vi "UHR-Fleezers Control (host) - 11.9c.vi"() -> ()   [LabVIEW 2014] (continued)
                  n307 = local read "Y RF Frequency Limits (MHz)"() -> (w501:T17)
                  n308 = local read "X RF Frequency Limits (MHz)"() -> (w502:T17)
                  n309 = local read "BD 2 Frequency 2 (MHz)"() -> (w508:dbl)
                  n310 = local read "BD 2 Frequency 3 (MHz)"() -> (w507:dbl)
                  n311 = local read "BD 1 Frequency 3 (MHz)"() -> (w509:dbl)
                  n312 = call "set RF board frequency - interlace.vi"("Board 2 Frequency Limits"=w501, "Board 1 Frequency Limits"=w502, "FPGA VI Reference In"=w494, "Board 2 Frequency 3 (MHz)"=w507, "Board 1 Frequency 3 (MHz)"=w509, "Board 2 Frequency 2 (MHz)"=w508, "Board 2 Frequency 1 (MHz)"=w505, "Board 1 Frequency 2 (MHz)"=w495, "Board 1 Frequency 1  (MHz)"=w506) -> ()  [unwired: 1 in, 2 out]
                }
                frame #1 {
                  n313 = And(x=w559, y=w556) -> (x .and. y?=w558:bool)
                  n314 = case "Only if were fishing and now formed tether" shown="True" w558 {
                    tunnel: w557 -> [w561 w576]
                    tunnel: [w560 w575] -> w555
                    tunnel: w554 -> [_ w571]
                    frame False {
                      n315 = local read "Fish"() -> (w560:bool)
                      n316 = case shown="False" w560 {
                        tunnel: w561 -> [w562 _]
                        frame False {
                          n317 = property on="BD 1 Frequency 1 (MHz)" class="DigNum (strict)"("Val(Sgnl)"=w562) -> ()  [unwired: 2 in, 2 out]
                        }
                        frame True {
                        }
                      }
                    }
                    frame True {
                      w575 = FALSE ("Fish for Tether")
                      n318 = call <vilib>:"Beep.vi"() -> ()  [unwired: 3 in, 9 out]
                      n319 = Number To Decimal String(number=w571, width (-)=i16 1) -> (decimal integer string=w569:string)
                      n320 = Concatenate Strings("Formed tether in ", w569, " attempt(s)." ("string")) -> (w566:string)
                      n321 = local read "Messages"() -> (w573:string)
                      n322 = local write "Fish"(w575) -> ()
                      n323 = call "Update messages.vi"("Message to add"=w566, "Old message string"=w573) -> ("New message string"=w572:string)
                      n324 = local write "Messages"(w572) -> ()
                      n325 = Get Date/Time In Seconds() -> (seconds since 1Jan1904=→"Time tether formed":timestamp)
                      n326 = local read "Flow ON\nduring cal?"() -> (w563:bool)
                      n327 = property on="Sample Channel\nFlow" class="Bool (strict)"("Val(Sgnl)"=w563) -> (error out=w564:errorcluster)  [unwired: 2 in, 1 out]
                      n328 = case shown="\"2\", \"3\", \"4\", \"5\", \"6\"" "Then..." {
                        selector: "Then..." -> [_ w579 _ _]
                        tunnel: w576 -> [w578 _ _ _]
                        tunnel: w564 -> [_ _ _ _]
                        frame "1", Default {
                          n329 = property on="BD 1 Frequency 1 (MHz)" class="DigNum (strict)"("Val(Sgnl)"=w578) -> ()  [unwired: 2 in, 2 out]
                        }
                        frame "2", "3", "4", "5", "6" {
                          n330 = flat-sequence {
                            tunnel: w579 -> [w585]
                            frame #0 {
                              n331 = local read "Flow ON\nduring cal?"() -> (w580:bool)
                              n332 = property on="Sample Channel\nFlow" class="Bool (strict)"("Val(Sgnl)"=w580) -> ()  [unwired: 2 in, 2 out]
                              n333 = property on="Trap D (MHz)" class="DigNum (strict)"("Val(Sgnl)"="Move to D 1 (MHz)") -> ()  [unwired: 2 in, 2 out]
                            }
                            frame #1 {
                              n334 = local read "Wait Before Save (s)"() -> (w582:u32)
                              n335 = Multiply(x=u32 1000 ("milliseconds to wait"), y=w582) -> (x*y=w584:u32)
                              n336 = Wait (ms)(milliseconds to wait=w584) -> ()  [unwired: 1 out]
                            }
                            frame #2 {
                              n337 = case shown="\"5\", \"6\"" w585 {
                                selector: w585 -> [w588 w598 _]
                                frame "3", "4" {
                                n338 = flat-sequence {
                                tunnel: w588 -> [w589]
                                tunnel: [w589] -> w586
                                tunnel: [w591] -> w587
                                tunnel: w586 -> [w591]
                                tunnel: w587 -> [w595]
                                frame #0 {
                                n339 = property on="Green ON/Interlacing" class="Bool (strict)"("Val(Sgnl)"=TRUE ("Value (Signaling)")) -> ()  [unwired: 2 in, 2 out]
                                }
                                frame #1 {
                                n340 = Multiply(x="Wait Before Save (s)", y=u32 1000 ("x")) -> (x*y=w593:u32)
                                n341 = Wait (ms)(milliseconds to wait=w593) -> ()  [unwired: 1 out]
                                }
                                frame #2 {
                                n342 = property on="Start Saving" class="Bool (strict)"("Value"=TRUE ("Start Saving")) -> ()  [unwired: 2 in, 2 out]
                                n343 = case shown="\"4\"" w595 {
                                frame Default {
                                }
                                frame "4" {
                                n344 = property on="Fl. Triggered..." class="Bool (strict)"("Val(Sgnl)"=TRUE ("Value (Signaling)")) -> ()  [unwired: 2 in, 2 out]
                                }
                                }
                                }
                                }
                                }
                                frame "5", "6" {
                                n345 = stacked-sequence {
                                tunnel: w598 -> [_ _ _ _ _ _ w610]
                                frame #0 {
                                n346 = Replace Array Subset(array=u32[] [0] ("Index Values"), new element="Raster Set\nUpon Tether", index=0) -> (w599:u32[])
                                n347 = property on="Saved AOD Raster Scan Parameter Sets" class="Arr (strict)"("Index Values"=w599) -> ()  [unwired: 2 in, 2 out]
                                }
                                frame #1 {
                                n348 = Wait (ms)(milliseconds to wait=u32 500) -> ()  [unwired: 1 out]
                                }
                                frame #2 {
                                n349 = property on="Load parameters" class="Bool (strict)"("Val(Sgnl)"=TRUE ("Value (Signaling)")) -> ()  [unwired: 2 in, 2 out]
                                n350 = case shown="True" "Green ON during\nraster?" {
                                frame False {
                                }
                                frame True {
                                n351 = property on="Green ON/Interlacing" class="Bool (strict)"("Val(Sgnl)"=TRUE ("Value (Signaling)")) -> ()  [unwired: 2 in, 2 out]
                                }
                                }
                                }
                                frame #3 {
                                n352 = Wait (ms)(milliseconds to wait=u32 500) -> ()  [unwired: 1 out]
                                }
                                frame #4 {
                                n353 = property on="Trap Raster Scan" class="Bool (strict)"("Val(Sgnl)"=TRUE ("Value (Signaling)")) -> ()  [unwired: 2 in, 2 out]
                                }
                                frame #5 {
                                n354 = Wait (ms)(milliseconds to wait=u32 2000) -> ()  [unwired: 1 out]
                                }
                                frame #6 {
                                n355 = flat-sequence {
                                tunnel: w610 -> [w617]
                                frame #0 {
                                n356 = while {
                                stop <- w613 stop-if-true
                                n357 = local read "Raster Scanning..."() -> (w612:bool)
                                n358 = local read "Saving..."() -> (w615:bool)
                                n359 = Wait (ms)(milliseconds to wait=u32 100) -> ()  [unwired: 1 out]
                                n360 = Not(x=w615) -> (.not. x?=w614:bool)
                                n361 = Not(x=w612) -> (.not. x?=w611:bool)
                                n362 = And(x=w614, y=w611) -> (x .and. y?=w613:bool)
                                }
                                }
                                frame #1 {
                                n363 = local read "Tether"() -> (w618:bool)
                                n364 = case shown="True" w618 {
                                tunnel: w617 -> [_ w620]
                                frame False {
                                n365 = property on="Fish" class="Bool (strict)"("Val(Sgnl)"="Fish again after \nraster break?") -> ()  [unwired: 2 in, 2 out]
                                }
                                frame True {
                                n366 = stacked-sequence {
                                tunnel: w620 -> [_ w624 _ _ _ _ _ _]
                                frame #0 {
                                n367 = property on="Trap D (MHz)" class="DigNum (strict)"("Val(Sgnl)"="Move to D 2 (MHz)") -> ()  [unwired: 2 in, 2 out]
                                n368 = case shown="True" "Flow ON after\ntether testing?" {
                                frame False {
                                }
                                frame True {
                                n369 = property on="Sample Channel\nFlow" class="Bool (strict)"("Val(Sgnl)"=TRUE ("Value (Signaling)")) -> ()  [unwired: 2 in, 2 out]
                                }
                                }
                                }
                                frame #1 {
                                n370 = flat-sequence {
                                tunnel: w624 -> [w625]
                                frame #0 {
                                n371 = case shown="\"6\"" w625 {
                                frame Default {
                                }
                                frame "6" {
                                n372 = flat-sequence {
                                frame #0 {
                                n373 = Wait (ms)(milliseconds to wait=u32 500) -> ()  [unwired: 1 out]
                                }
                                frame #1 {
                                n374 = property on="Green ON/Interlacing" class="Bool (strict)"("Val(Sgnl)"=TRUE ("Green Laser ON/Interlacing")) -> ()  [unwired: 2 in, 2 out]
                                }
                                }
                                }
                                }
                                }
                                frame #1 {
                                n375 = case shown="True" "Save at end (5, 6)" {
                                selector: "Save at end (5, 6)" -> [_ w629]
                                frame False {
                                }
                                frame True {
                                n376 = flat-sequence {
                                tunnel: w629 -> [w631]
                                frame #0 {
                                n377 = Wait (ms)(milliseconds to wait=u32 500) -> ()  [unwired: 1 out]
                                }
                                frame #1 {
                                n378 = local write "Start Saving"(w631) -> ()
                                }
                                }
                                }
                                }
                                }
                                }
                                }
                                frame #2 {
                                n379 = local read "Bead Sep. Int. Time (s)"() -> (w634:dbl)
                                n380 = Multiply(x=w634, y=1000.0) -> (x*y=w633:dbl)
                                n381 = Wait (ms)(milliseconds to wait=w633) -> ()  [unwired: 1 out]
                                }
                                frame #3 {
                                n382 = property on="Remove Offset" class="Bool (strict)"("Val(Sgnl)"=TRUE ("Value (Signaling)")) -> ()  [unwired: 2 in, 2 out]
                                }
                                frame #4 {
                                n383 = property on="Read FX file" class="Bool (strict)"("Val(Sgnl)"=TRUE ("Value (Signaling)")) -> ()  [unwired: 2 in, 2 out]
                                }
                                frame #5 {
                                n384 = Wait (ms)(milliseconds to wait=u32 300) -> ()  [unwired: 1 out]
                                }
                                frame #6 {
                                n385 = local read "Bad fit error"() -> (w643:dbl)
                                n386 = local read "Fit offset"() -> (w646:dbl)
                                n387 = Greater Or Equal?(x=w643, y="Bad fit thresh") -> (x >= y?=→"Bad fit":bool)
                                n388 = Greater Or Equal?(x=w646, y="Fit offset thresh") -> (x >= y?=→"Multiple tether":bool)
                                n389 = local read "Hyst. error"() -> (w640:dbl)
                                n390 = Greater Or Equal?(x=w640, y="Hysteresis thresh") -> (x >= y?=→"Hysteresis":bool)
                                }
                                frame #7 {
                                w651 = 0
                                n391 = local read "Bad fit error"() -> (w653:dbl)
                                n392 = local read "Hyst. error"() -> (w652:dbl)
                                n393 = local read "Fit offset"() -> (w654:dbl)
                                n394 = local read "Multiple tether"() -> (w660:bool)
                                n395 = local read "Hysteresis"() -> (w658:bool)
                                n396 = local read "Bad fit"() -> (w659:bool)
                                n397 = Not(x=w658) -> (.not. x?=w650:bool)
                                n398 = Not(x=w659) -> (.not. x?=w656:bool)
                                n399 = Greater?(x=w654, y=w651) -> (0:w649:bool)
                                n400 = Greater?(x=w653, y=w651) -> (0:w648:bool)
                                n401 = Greater?(x=w652, y=w651) -> (0:w647:bool)
                                n402 = Not(x=w660) -> (.not. x?=w657:bool)
                                n403 = Compound Arithmetic op=AND(w657, w656, w650, w649, w648, w647) -> (w655:bool)
                                "Good tether" <- w655
                                n404 = case shown="True" w655 {
                                frame False {
                                }
                                frame True {
                                n405 = call <vilib>:"Beep.vi"("use system alert? (T)"=FALSE, "duration (msec)"=u32 200, "frequency (Hz)"=u32 2000) -> ()  [unwired: 9 in]
                                }
                                }
                                }
                                }
                                }
                                }
                                }
                                }
                                }
                                }
                                }
                                frame "2", Default {
                                }
                              }
                            }
                            frame #3 {
                              n406 = local read "Multiple tether"() -> (w666:bool)
                              n407 = And(x="Break multiple", y=w666) -> (x .and. y?=w664:bool)
                              n408 = case shown="True" w664 {
                                frame False {
                                }
                                frame True {
                                n409 = stacked-sequence {
                                frame #0 {
                                n410 = property on="Trap D (MHz)" class="DigNum (strict)"("Val(Sgnl)"="Trap D to \nbreak (MHz)") -> ()  [unwired: 2 in, 2 out]
                                }
                                frame #1 {
                                n411 = case shown="True" "Fish after\nmultiple break" {
                                frame False {
                                }
                                frame True {
                                n412 = while {
                                stop <- w671 stop-if-true
                                n413 = local read "Multiple tether"() -> (w673:bool)
                                n414 = local read "Fish"() -> (w670:bool)
                                n415 = local read "Stop All"() -> (w669:bool)
                                n416 = Wait (ms)(milliseconds to wait=u32 100) -> ()  [unwired: 1 out]
                                n417 = Not(x=w673) -> (.not. x?=w672:bool)
                                n418 = Compound Arithmetic op=OR(w669, w672, w670) -> (w671:bool)
                                }
                                }
                                }
                                }
                                frame #2 {
                                n419 = local read "Fish after\nmultiple break"() -> (w678:bool)
                                n420 = local read "Stage Moving"() -> (w677:bool)
                                n421 = Not(x=w677) -> (.not. x?=w675:bool)
                                n422 = And(x=w678, y=w675) -> (x .and. y?=w676:bool)
                                n423 = property on="Fish" class="Bool (strict)"("Val(Sgnl)"=w676) -> ()  [unwired: 2 in, 2 out]
                                }
                                }
                                }
                              }
                            }
                            frame #4 {
                              n424 = local read "Bad fit"() -> (w680:bool)
                              n425 = And(x="Break bad fit", y=w680) -> (x .and. y?=w679:bool)
                              n426 = case shown="True" w679 {
                                frame False {
                                }
                                frame True {
                                n427 = stacked-sequence {
                                frame #0 {
                                n428 = local read "Trap D to \nbreak (MHz)"() -> (w682:dbl)
                                n429 = property on="Trap D (MHz)" class="DigNum (strict)"("Val(Sgnl)"=w682) -> ()  [unwired: 2 in, 2 out]
                                }
                                frame #1 {
                                n430 = case shown="True" "Fish after\nbad fit break?" {
                                frame False {
                                }
                                frame True {
                                n431 = while {
                                stop <- w686 stop-if-true
                                n432 = local read "Stop All"() -> (w684:bool)
                                n433 = local read "Bad fit"() -> (w685:bool)
                                n434 = local read "Fish"() -> (w687:bool)
                                n435 = Not(x=w685) -> (.not. x?=w688:bool)
                                n436 = Wait (ms)(milliseconds to wait=u32 100) -> ()  [unwired: 1 out]
                                n437 = Compound Arithmetic op=OR(w684, w688, w687) -> (w686:bool)
                                }
                                }
                                }
                                }
                                frame #2 {
                                n438 = local read "Fish after\nbad fit break?"() -> (w690:bool)
                                n439 = local read "Stage Moving"() -> (w693:bool)
                                n440 = Not(x=w693) -> (.not. x?=w692:bool)
                                n441 = And(x=w690, y=w692) -> (x .and. y?=w691:bool)
                                n442 = property on="Fish" class="Bool (strict)"("Val(Sgnl)"=w691) -> ()  [unwired: 2 in, 2 out]
                                }
                                }
                                }
                              }
                            }
                            frame #5 {
                              n443 = local read "Hysteresis"() -> (w695:bool)
                              n444 = And(x="Break hyst", y=w695) -> (x .and. y?=w694:bool)
                              n445 = case shown="True" w694 {
                                frame False {
                                }
                                frame True {
                                n446 = stacked-sequence {
                                frame #0 {
                                n447 = local read "Trap D to \nbreak (MHz)"() -> (w697:dbl)
                                n448 = property on="Trap D (MHz)" class="DigNum (strict)"("Val(Sgnl)"=w697) -> ()  [unwired: 2 in, 2 out]
                                }
                                frame #1 {
                                n449 = case shown="True" "Fish ater hyst?" {
                                frame False {
                                }
                                frame True {
                                n450 = while {
                                stop <- w703 stop-if-true
                                n451 = local read "Hysteresis"() -> (w702:bool)
                                n452 = local read "Stop All"() -> (w699:bool)
                                n453 = local read "Fish"() -> (w700:bool)
                                n454 = Wait (ms)(milliseconds to wait=u32 100) -> ()  [unwired: 1 out]
                                n455 = Not(x=w702) -> (.not. x?=w701:bool)
                                n456 = Compound Arithmetic op=OR(w699, w701, w700) -> (w703:bool)
                                }
                                }
                                }
                                }
                                frame #2 {
                                n457 = local read "Fish ater hyst?"() -> (w708:bool)
                                n458 = local read "Stage Moving"() -> (w707:bool)
                                n459 = Not(x=w707) -> (.not. x?=w706:bool)
                                n460 = And(x=w708, y=w706) -> (x .and. y?=w705:bool)
                                n461 = property on="Fish" class="Bool (strict)"("Val(Sgnl)"=w705) -> ()  [unwired: 2 in, 2 out]
                                }
                                }
                                }
                              }
                            }
                            frame #6 {
                              n462 = local read "Good tether"() -> (w709:bool)
                              n463 = case shown="True" w709 {
                                frame False {
                                }
                                frame True {
                                n464 = case shown="\"1\"" "If good, then:" {
                                frame "0", Default {
                                }
                                frame "1" {
                                n465 = property on="Force FB Script" class="Bool (strict)"("Val(Sgnl)"=TRUE ("Value (Signaling)")) -> ()  [unwired: 2 in, 2 out]
                                }
                                }
                                }
                              }
                            }
                          }
                        }
                        frame "7" {
                          n466 = property on="Force FB Script" class="Bool (strict)"("Val(Sgnl)"=TRUE ("Value (Signaling)")) -> ()  [unwired: 2 in, 2 out]
                        }
                        frame "8" {
                          n467 = property on="Fixed Traps Script" class="Bool (strict)"("Val(Sgnl)"=TRUE ("Value (Signaling)")) -> ()  [unwired: 2 in, 2 out]
                        }
                      }
                      "Tether" <- "Tether Alarm?"
                    }
                  }
                }
                frame #2 {
                  n468 = local read "Oscillate Set 1"() -> (w719:bool)
                  n469 = local read "Stop All"() -> (w717:bool)
                  n470 = Or(x=w719, y=w714) -> (x .or. y?=w716:bool)
                  n471 = Not(x=w716) -> (.not. x?=w718:bool)
                  n472 = Compound Arithmetic op=OR(w717, w718) -> (w715:bool)
                }
              }
              n473 = node-c288() -> ()  [unwired: 2 out]
            }
            n474 = node-c288(w469) -> ()  [unwired: 1 out]
          }
        }
      }
      event "Fl. Triggered...": Value Change {
        n475 = event-data() -> ()  [unwired: 7 out]
        n476 = case shown="True" "Fl. Triggered..." {
          frame False {
          }
          frame True {
            n477 = node-c288() -> (w730:T22)  [unwired: 4 out]
            n478 = timed-loop {
              timing: w730 -> [_]
              timing-out: [_] -> w729
              tunnel: "Action" -> [w738]
              shift-right: [w735] -> _
              shift-left: u8 255 -> [w737]
              shift-right: [w732] -> _
              shift-left: 255 -> [w734]
              stop <- w731 stop-if-true
              # "Reset confocal spot"
              n479 = node-c288() -> ()  [unwired: 2 out]
              n480 = flat-sequence {
                tunnel: w738 -> [w758]
                tunnel: w737 -> [w757]
                tunnel: [w756] -> w736
                tunnel: w734 -> [w743]
                tunnel: [w742] -> w733
                tunnel: [w1142] -> w731
                tunnel: w736 -> [w1141]
                tunnel: [w1141] -> w735
                tunnel: [w1140] -> w732
                tunnel: w733 -> [w1140]
                frame #0 {
                  n481 = local read "Delta Fl. 2"() -> (w755:dbl)
                  n482 = local read "Delta Fl. 1"() -> (w750:dbl)
                  n483 = Multiply(x="Fl. D Thresh. (kHz)", y=1000.0) -> (x*y=w745:dbl)
                  n484 = Select(t=w750, s="APD to Watch", f=w755) -> (s? t:f=w746:dbl)
                  n485 = Greater?(x=w746, y=w745) -> (0:w751:bool)
                  n486 = Or(x="Force Yank", y=w751) -> (x .or. y?=w749:bool)
                  n487 = And(x=w749, y="Yank when?") -> (x .and. y?=w747:bool)
                  n488 = case shown="False" w747 {
                    tunnel: w758 -> [w761 w964]
                    tunnel: w757 -> [w763 w960]
                    tunnel: [w763 w958] -> w756
                    tunnel: w746 -> [w769 _]
                    tunnel: w745 -> [w768 _]
                    tunnel: "Force Yank" -> [w766 _]
                    tunnel: w743 -> [w765 w957]
                    tunnel: [w764 w957] -> w742
                    frame False {
                      n489 = Negate(x=w768) -> (-x=w760:dbl)
                      n490 = local write "Fl. High"(TRUE ("Fl. High")) -> ()
                      n491 = Less?(x=w769, y=w760) -> (x < y?=w767:bool)
                      n492 = Or(x=w766, y=w767) -> (x .or. y?=w762:bool)
                      n493 = case shown="True" w762 {
                        tunnel: w765 -> [w770 w780]
                        tunnel: [w770 w779] -> w764
                        tunnel: w761 -> [_ w778]
                        frame False {
                        }
                        frame True {
                          n494 = flat-sequence {
                            tunnel: w780 -> [w786]
                            tunnel: w778 -> [w783]
                            tunnel: [w785] -> w777
                            tunnel: [w784] -> w776
                            tunnel: [w783] -> w775
                            tunnel: w774 -> [w782]
                            tunnel: [w782] -> w773
                            tunnel: w772 -> [w781]
                            tunnel: [w781] -> w771
                            tunnel: [w858] -> w779
                            tunnel: w777 -> [w858]
                            tunnel: w776 -> [w857]
                            tunnel: w775 -> [w856]
                            tunnel: w773 -> [w855]
                            tunnel: w771 -> [w854]
                            frame #0 {
                              n495 = call <vilib>:"Beep.vi"() -> ()  [unwired: 12 in]
                              n496 = local write "Waiting"(FALSE ("Waiting")) -> ()
                              n497 = Increment(x=w786) -> (x+1=w785:i32)
                              n498 = case shown="\"Yank\"" w783 {
                                tunnel: w785 -> [_ w791 _]
                                frame "Alarm", Default {
                                }
                                frame "Yank" {
                                n499 = flat-sequence {
                                tunnel: w791 -> [w794]
                                tunnel: [w793] -> w790
                                tunnel: [w792] -> w789
                                tunnel: w790 -> [w804]
                                tunnel: w789 -> [w805]
                                frame #0 {
                                n500 = local read "Yank Delay (s)"() -> (w797:dbl)
                                n501 = local read "N Array El"() -> (w792:u8)
                                n502 = Quotient & Remainder(x=w794, y=w792) -> (x-y*floor(x/y)=w793:i32)  [unwired: 1 out]
                                n503 = Multiply(x=w797, y=1000.0) -> (x*y=w795:dbl)
                                n504 = Wait (ms)(milliseconds to wait=w795) -> ()  [unwired: 1 out]
                                }
                                frame #1 {
                                n505 = local read "Yank to which?"() -> (w799:bool)
                                n506 = local read "Random Choice"() -> (w809:bool)
                                n507 = local read "Yank to Trap D (MHz)"() -> (w802:dbl[])
                                n508 = local read "Yank to SP"() -> (w803:dbl[])
                                n509 = Random Number (0-1)() -> (number: 0 to 1=w808:dbl)
                                n510 = Multiply(x=w805, y=w808) -> (x*y=w807:dbl)
                                n511 = Round Toward -Infinity(1:w807) -> (0:w806:dbl)
                                n512 = Select(t=w806, s=w809, f=w804) -> (s? t:f=w800:dbl)
                                n513 = Select(t=w802, s=w799, f=w803) -> (s? t:f=w801:dbl[])
                                n514 = Index Array(array=w801, index=w800) -> (element=w798:dbl)
                                n515 = case shown="False" w799 {
                                tunnel: w798 -> [w810 w838]
                                frame False {
                                n516 = flat-sequence {
                                tunnel: w810 -> [w811]
                                frame #0 {
                                n517 = property on="Trap Pos FB SP" class="DigNum (strict)"("Val(Sgnl)"=w811) -> ()  [unwired: 2 in, 2 out]
                                }
                                frame #1 {
                                n518 = Wait (ms)(milliseconds to wait=u32 700) -> ()  [unwired: 1 out]
                                }
                                frame #2 {
                                n519 = local read "Action (%)"() -> (w816:dbl)
                                n520 = Absolute Value(x=w816) -> (abs(x)=w815:dbl)
                                n521 = Greater?(x=w815, y=70.0) -> (0:w813:bool)
                                n522 = property on="Remove Action Offset" class="Bool (strict)"("Val(Sgnl)"=w813) -> ()  [unwired: 2 in, 2 out]
                                }
                                frame #3 {
                                n523 = for {
                                N: 4 -> [_]
                                n524 = flat-sequence {
                                frame #0 {
                                n525 = Wait (ms)(milliseconds to wait=u32 500) -> ()  [unwired: 1 out]
                                }
                                frame #1 {
                                n526 = local read "Action (%)"() -> (w822:dbl)
                                n527 = Absolute Value(x=w822) -> (abs(x)=w821:dbl)
                                n528 = Greater?(x=w821, y=70.0) -> (0:w819:bool)
                                n529 = property on="Remove Action Offset" class="Bool (strict)"("Val(Sgnl)"=w819) -> ()  [unwired: 2 in, 2 out]
                                }
                                }
                                }
                                }
                                frame #4 {
                                n530 = Wait (ms)(milliseconds to wait=u32 500) -> ()  [unwired: 1 out]
                                }
                                frame #5 {
                                n531 = local read "Mean"() -> (w830:dbl)
                                n532 = Greater?(x=w830, y=11.0) -> (0:w824:bool)
                                n533 = Not(x=w824) -> (.not. x?=w825:bool)
                                n534 = And(x=w825, y="Shift confocal") -> (x .and. y?=w827:bool)
                                n535 = And(x=w824, y="Shift confocal") -> (x .and. y?=w828:bool)
                                n536 = case shown="True" w828 {
                                frame False {
                                }
                                frame True {
                                n537 = local read "Confocal Y 2 (V)"() -> (w834:dbl)
                                n538 = local read "Confocal X 2 (V)"() -> (w833:dbl)
                                n539 = property on="AO1" class="Slide (strict)"("Val(Sgnl)"=w834) -> ()  [unwired: 2 in, 2 out]
                                n540 = property on="AO2" class="Slide (strict)"("Val(Sgnl)"=w833) -> ()  [unwired: 2 in, 2 out]
                                }
                                }
                                n541 = case shown="True" w827 {
                                frame False {
                                }
                                frame True {
                                n542 = local read "Confocal Y 1 (V)"() -> (w832:dbl)
                                n543 = local read "Confocal X 1 (V)"() -> (w831:dbl)
                                n544 = property on="AO1" class="Slide (strict)"("Val(Sgnl)"=w832) -> ()  [unwired: 2 in, 2 out]
                                n545 = property on="AO2" class="Slide (strict)"("Val(Sgnl)"=w831) -> ()  [unwired: 2 in, 2 out]
                                }
                                }
                                }
                                frame #6 {
                                n546 = Wait (ms)(milliseconds to wait=u32 1500) -> ()  [unwired: 1 out]
                                }
                                frame #7 {
                                n547 = property on="Rem fb disp offset" class="Bool (strict)"("Val(Sgnl)"=TRUE ("Value (Signaling)")) -> ()  [unwired: 2 in, 2 out]
                                n548 = property on="Remove Offset" class="Bool (strict)"("Val(Sgnl)"=TRUE ("Value (Signaling)")) -> ()  [unwired: 2 in, 2 out]
                                }
                                }
                                }
                                frame True {
                                n549 = flat-sequence {
                                tunnel: w838 -> [w839]
                                frame #0 {
                                n550 = property on="Trap D (MHz)" class="DigNum (strict)"("Val(Sgnl)"=w839) -> ()  [unwired: 2 in, 2 out]
                                }
                                frame #1 {
                                n551 = Wait (ms)(milliseconds to wait=u32 500) -> ()  [unwired: 1 out]
                                }
                                frame #2 {
                                n552 = local read "Shift confocal"() -> (w845:bool)
                                n553 = local read "Mean"() -> (w847:dbl)
                                n554 = Greater?(x=w847, y=11.0) -> (0:w844:bool)
                                n555 = Not(x=w844) -> (.not. x?=w843:bool)
                                n556 = And(x=w843, y=w845) -> (x .and. y?=w841:bool)
                                n557 = And(x=w844, y=w845) -> (x .and. y?=w842:bool)
                                n558 = case shown="True" w842 {
                                frame False {
                                }
                                frame True {
                                n559 = local read "Confocal Y 2 (V)"() -> (w851:dbl)
                                n560 = local read "Confocal X 2 (V)"() -> (w850:dbl)
                                n561 = property on="AO2" class="Slide (strict)"("Val(Sgnl)"=w850) -> ()  [unwired: 2 in, 2 out]
                                n562 = property on="AO1" class="Slide (strict)"("Val(Sgnl)"=w851) -> ()  [unwired: 2 in, 2 out]
                                }
                                }
                                n563 = case shown="True" w841 {
                                frame False {
                                }
                                frame True {
                                n564 = local read "Confocal X 1 (V)"() -> (w848:dbl)
                                n565 = local read "Confocal Y 1 (V)"() -> (w849:dbl)
                                n566 = property on="AO2" class="Slide (strict)"("Val(Sgnl)"=w848) -> ()  [unwired: 2 in, 2 out]
                                n567 = property on="AO1" class="Slide (strict)"("Val(Sgnl)"=w849) -> ()  [unwired: 2 in, 2 out]
                                }
                                }
                                }
                                }
                                }
                                }
                                }
                                }
                                }
                                frame "Image" {
                                n568 = property on="Confocal\nImage" class="Bool (strict)"("Val(Sgnl)"=TRUE ("Value (Signaling)")) -> ()  [unwired: 2 in, 2 out]
                                }
                              }
                              n569 = local write "Fl. High"(FALSE ("Fl. High")) -> ()
                              n570 = local read "Time (s)"() -> (w784:dbl)
                            }
                            frame #1 {
                              n571 = case shown="True" "Auto F Reset" {
                                tunnel: w857 -> [_ w862]
                                tunnel: w856 -> [_ w861]
                                tunnel: w855 -> [_ w860]
                                tunnel: w854 -> [_ w859]
                                frame False {
                                }
                                frame True {
                                n572 = node-c288() -> (w864:T22)  [unwired: 4 in]
                                n573 = timed-loop {
                                timing: w864 -> [_]
                                timing-out: [_] -> w863
                                tunnel: w862 -> [w869]
                                tunnel: w861 -> [w868]
                                tunnel: w860 -> [w867]
                                tunnel: w859 -> [w866]
                                stop <- w865 stop-if-true
                                n574 = node-c288() -> ()  [unwired: 1 in, 1 out]
                                n575 = local read "APD to Watch"() -> (w879:bool)
                                n576 = local read "Fl. D Thresh. (kHz)"() -> (w878:dbl)
                                n577 = local read "Delta Fl. 1"() -> (w880:dbl)
                                n578 = local read "Delta Fl. 2"() -> (w881:dbl)
                                n579 = local read "Fl. Triggered..."() -> (w872:bool)
                                n580 = local read "Stop All"() -> (w873:bool)
                                n581 = local read "Reset Force"() -> (w871:bool)
                                n582 = Multiply(x=w878, y=1000.0) -> (x*y=w876:dbl)
                                n583 = Not(x=w872) -> (.not. x?=w870:bool)
                                n584 = Select(t=w880, s=w879, f=w881) -> (s? t:f=w875:dbl)
                                n585 = Greater?(x=w875, y=w876) -> (0:w874:bool)
                                n586 = Compound Arithmetic op=OR(w874, w873, w870, w871) -> (w865:bool)
                                n587 = case shown="True" w865 {
                                tunnel: w869 -> [_ w885]
                                tunnel: w868 -> [_ w889]
                                tunnel: w867 -> [_ w888]
                                tunnel: w866 -> [_ w887]
                                frame False {
                                }
                                frame True {
                                n588 = case shown="\"Yank\"" w889 {
                                tunnel: w888 -> [_ w899]
                                tunnel: w887 -> [_ w897]
                                frame "Image", Default {
                                }
                                frame "Yank" {
                                n589 = flat-sequence {
                                tunnel: [w902] -> w900
                                tunnel: w899 -> [w902]
                                tunnel: [w901] -> w898
                                tunnel: w897 -> [w901]
                                tunnel: w900 -> [w908]
                                tunnel: w898 -> [w906]
                                frame #0 {
                                n590 = local read "Yank Delay (s)"() -> (w905:dbl)
                                n591 = Multiply(x=w905, y=1000.0) -> (x*y=w903:dbl)
                                n592 = Wait (ms)(milliseconds to wait=w903) -> ()  [unwired: 1 out]
                                }
                                frame #1 {
                                n593 = local read "Yank to which?"() -> (w907:bool)
                                n594 = case shown="False" w907 {
                                tunnel: w908 -> [_ w937]
                                tunnel: w906 -> [w909 _]
                                frame False {
                                n595 = flat-sequence {
                                tunnel: w909 -> [w910]
                                frame #0 {
                                n596 = property on="Trap Pos FB SP" class="DigNum (strict)"("Val(Sgnl)"=w910) -> ()  [unwired: 2 in, 2 out]
                                }
                                frame #1 {
                                n597 = Wait (ms)(milliseconds to wait=u32 700) -> ()  [unwired: 1 out]
                                }
                                frame #2 {
                                n598 = local read "Action (%)"() -> (w915:dbl)
                                n599 = Absolute Value(x=w915) -> (abs(x)=w914:dbl)
                                n600 = Greater?(x=w914, y=70.0) -> (0:w912:bool)
                                n601 = property on="Remove Action Offset" class="Bool (strict)"("Val(Sgnl)"=w912) -> ()  [unwired: 2 in, 2 out]
                                }
                                frame #3 {
                                n602 = for {
                                N: 4 -> [_]
                                n603 = flat-sequence {
                                frame #0 {
                                n604 = Wait (ms)(milliseconds to wait=u32 500) -> ()  [unwired: 1 out]
                                }
                                frame #1 {
                                n605 = local read "Action (%)"() -> (w921:dbl)
                                n606 = Absolute Value(x=w921) -> (abs(x)=w920:dbl)
                                n607 = Greater?(x=w920, y=70.0) -> (0:w918:bool)
                                n608 = property on="Remove Action Offset" class="Bool (strict)"("Val(Sgnl)"=w918) -> ()  [unwired: 2 in, 2 out]
                                }
                                }
                                }
                                }
                                frame #4 {
                                n609 = Wait (ms)(milliseconds to wait=u32 500) -> ()  [unwired: 1 out]
                                }
                                frame #5 {
                                n610 = local read "Shift confocal"() -> (w926:bool)
                                n611 = local read "Mean"() -> (w929:dbl)
                                n612 = Greater?(x=w929, y=11.0) -> (0:w925:bool)
                                n613 = Not(x=w925) -> (.not. x?=w924:bool)
                                n614 = And(x=w925, y=w926) -> (x .and. y?=w927:bool)
                                n615 = And(x=w924, y=w926) -> (x .and. y?=w923:bool)
                                n616 = case shown="True" w927 {
                                frame False {
                                }
                                frame True {
                                n617 = local read "Confocal X 2 (V)"() -> (w932:dbl)
                                n618 = local read "Confocal Y 2 (V)"() -> (w933:dbl)
                                n619 = property on="AO2" class="Slide (strict)"("Val(Sgnl)"=w932) -> ()  [unwired: 2 in, 2 out]
                                n620 = property on="AO1" class="Slide (strict)"("Val(Sgnl)"=w933) -> ()  [unwired: 2 in, 2 out]
                                }
                                }
                                n621 = case shown="True" w923 {
                                frame False {
                                }
                                frame True {
                                n622 = local read "Confocal Y 1 (V)"() -> (w931:dbl)
                                n623 = local read "Confocal X 1 (V)"() -> (w930:dbl)
                                n624 = property on="AO1" class="Slide (strict)"("Val(Sgnl)"=w931) -> ()  [unwired: 2 in, 2 out]
                                n625 = property on="AO2" class="Slide (strict)"("Val(Sgnl)"=w930) -> ()  [unwired: 2 in, 2 out]
                                }
                                }
                                }
                                frame #6 {
                                n626 = Wait (ms)(milliseconds to wait=u32 1500) -> ()  [unwired: 1 out]
                                }
                                frame #7 {
                                n627 = property on="Remove Offset" class="Bool (strict)"("Val(Sgnl)"=TRUE ("Value (Signaling)")) -> ()  [unwired: 2 in, 2 out]
                                n628 = property on="Rem fb disp offset" class="Bool (strict)"("Val(Sgnl)"=TRUE ("Value (Signaling)")) -> ()  [unwired: 2 in, 2 out]
                                }
                                }
                                }
                                frame True {
                                n629 = flat-sequence {
                                tunnel: w937 -> [w938]
                                frame #0 {
                                n630 = property on="Trap D (MHz)" class="DigNum (strict)"("Val(Sgnl)"=w938) -> ()  [unwired: 2 in, 2 out]
                                }
                                frame #1 {
                                n631 = Wait (ms)(milliseconds to wait=u32 500) -> ()  [unwired: 1 out]
                                }
                                frame #2 {
                                n632 = local read "Shift confocal"() -> (w944:bool)
                                n633 = local read "Mean"() -> (w945:dbl)
                                n634 = Greater?(x=w945, y=11.0) -> (0:w943:bool)
                                n635 = And(x=w943, y=w944) -> (x .and. y?=w941:bool)
                                n636 = Not(x=w943) -> (.not. x?=w942:bool)
                                n637 = And(x=w942, y=w944) -> (x .and. y?=w940:bool)
                                n638 = case shown="True" w941 {
                                frame False {
                                }
                                frame True {
                                n639 = local read "Confocal Y 2 (V)"() -> (w950:dbl)
                                n640 = local read "Confocal X 2 (V)"() -> (w949:dbl)
                                n641 = property on="AO1" class="Slide (strict)"("Val(Sgnl)"=w950) -> ()  [unwired: 2 in, 2 out]
                                n642 = property on="AO2" class="Slide (strict)"("Val(Sgnl)"=w949) -> ()  [unwired: 2 in, 2 out]
                                }
                                }
                                n643 = case shown="True" w940 {
                                frame False {
                                }
                                frame True {
                                n644 = local read "Confocal Y 1 (V)"() -> (w948:dbl)
                                n645 = local read "Confocal X 1 (V)"() -> (w947:dbl)
                                n646 = property on="AO2" class="Slide (strict)"("Val(Sgnl)"=w947) -> ()  [unwired: 2 in, 2 out]
                                n647 = property on="AO1" class="Slide (strict)"("Val(Sgnl)"=w948) -> ()  [unwired: 2 in, 2 out]
                                }
                                }
                                }
                                }
                                }
                                }
                                }
                                }
                                }
                                }
                                n648 = local read "Time (s)"() -> (w884:dbl)
                                n649 = Subtract(x=w885, y=w884) -> (x-y=w896:dbl)
                                n650 = Number To Decimal String(number=w896, width (-)=i16 0) -> (decimal integer string=w894:string)
                                n651 = Concatenate Strings(w894, " s fluorescence event") -> (w891:string)
                                n652 = local read "Messages"() -> (w892:string)
                                n653 = local write "Duration (s)"(w896) -> ()
                                n654 = call "Update messages.vi"("Message to add"=w891, "Old message string"=w892) -> ("New message string"=w890:string)
                                n655 = local write "Messages"(w890) -> ()
                                n656 = call <vilib>:"Beep.vi"() -> ()  [unwired: 12 in]
                                n657 = local write "Reset Force"(FALSE ("Force Reset")) -> ()
                                n658 = local write "Fl. High"(TRUE ("Fl. High")) -> ()
                                n659 = local write "Waiting"(TRUE ("Waiting")) -> ()
                                }
                                }
                                n660 = node-c288() -> ()  [unwired: 1 in, 1 out]
                                }
                                n661 = node-c288(w863) -> ()  [unwired: 1 out]
                                }
                              }
                            }
                          }
                          n662 = local read "Trap Pos FB SP"() -> (w772:fxp<+/-,16,1>)
                          n663 = local read "Trap D (MHz)"() -> (w774:dbl)
                        }
                      }
                    }
                    frame True {
                      n664 = flat-sequence {
                        tunnel: w961 -> [w971]
                        tunnel: [w971] -> w965
                        tunnel: w964 -> [w970]
                        tunnel: [w970] -> w963
                        tunnel: [w969] -> w962
                        tunnel: w960 -> [w968]
                        tunnel: [w967] -> w959
                        tunnel: w956 -> [w966]
                        tunnel: [w966] -> w955
                        tunnel: w965 -> [w1043]
                        tunnel: w963 -> [w1042]
                        tunnel: w962 -> [w1041]
                        tunnel: w959 -> [w1040]
                        tunnel: w955 -> [w1039]
                        tunnel: [w1040] -> w958
                        frame #0 {
                          n665 = call <vilib>:"Beep.vi"() -> ()  [unwired: 3 in, 9 out]
                          n666 = local write "Waiting"(FALSE ("Waiting")) -> ()
                          n667 = Increment(x=w968) -> (x+1=w967:u8)
                          n668 = case shown="\"Image\"" w970 {
                            tunnel: w967 -> [_ _ w977 _]
                            frame "Image" {
                              n669 = property on="Confocal\nImage" class="Bool (strict)"("Val(Sgnl)"=TRUE ("Value (Signaling)")) -> ()  [unwired: 2 in, 2 out]
                            }
                            frame "Alarm", Default {
                            }
                            frame "Yank" {
